vi "Run Bfr Rx - CachedSize - Flush Cache.vi"(8 "error in (no error)":errorcluster, 11 "Cached Buffer in":T1 {"Cache Buffer" format="%016x"}) -> (0 "error out":errorcluster, 3 "Cached Buffer out":T1 {"Cache Buffer" format="%016x"})   [LabVIEW 2016, in "UDP-Custom-Device Engine.lvlib"]
uses:
  UDP-Custom-Device Engine.lvlib
  Types/Engine - Buffered Rx Cached Buffer.ctl
  <vilib>/NI Veristand/VeriStand Data/Pointer Operations/Pointer.Write (1D U8).vi
  <vilib>/NI Veristand/VeriStand Data/VeriStand Data.lvlib
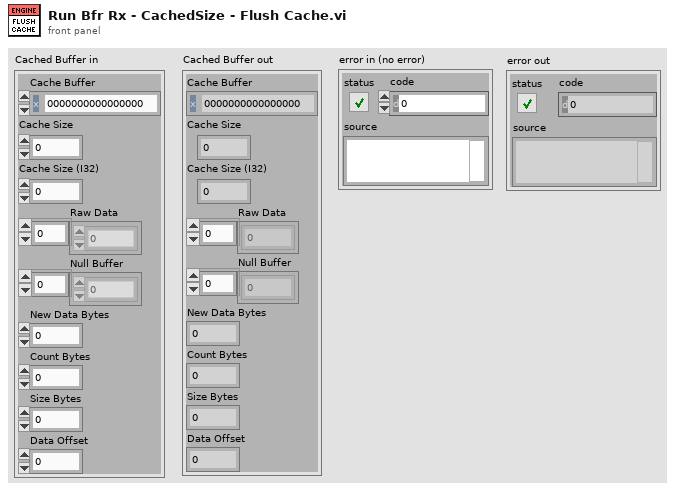
[diagram p1: front panel]
types:
  T1 = typedef "UDP-Custom-Device Engine.lvlib/Engine - Buffered Rx Cached Buffer.ctl" = cluster{"Cache Buffer":u64, "Cache Size":u64, "Cache Size (I32)":i32, "Raw Data":u8[], "Null Buffer":u8[], "New Data Bytes":u64, "Count Bytes":u64, "Size Bytes":u64, "Data Offset":u64}
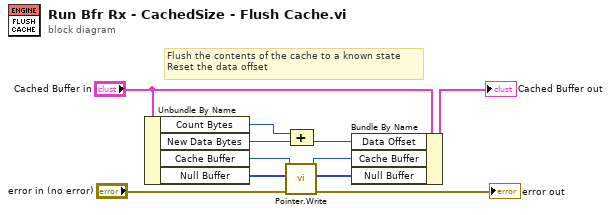
[diagram p0: block diagram]
diagram:
  # "Flush the contents of the cache to a known state\nReset the data offset"
  n1 = Unbundle By Name("Cached Buffer in") -> ("Count Bytes"=w2:u64, "New Data Bytes"=w3:u64, "Cache Buffer"=w9:u64, "Null Buffer"=w10:u8[])
  n2 = call-poly <vilib>:"Pointer.Write.vi"("error in (no error)"="error in (no error)", "values"=w10, "pointer in"=w9) -> ("error out"=→"error out":errorcluster, "values out"=w7:u8[], "pointer out"=w6:u64)  [unwired: 6 in]
  n3 = Compound Arithmetic op=ADD(w2, w3) -> (w1:u64)
  n4 = Bundle By Name(cluster="Cached Buffer in", "Data Offset"=w1, "Cache Buffer"=w6, "Null Buffer"=w7) -> (→"Cached Buffer out":T1)
